vi "PostCopyScripting.vi"(10 "MetaDataObj":refnum<class "MetaDataObj.lvclass">, 11 "User Project":refnum<vi>) -> ()   [LabVIEW 2021, in "myRIOMetaDataObj.lvclass"]
uses:
  myRIOMetaDataObj.lvclass
  <resource>/dialog/NewProjectWizard/MetaDataObj/MetaDataObj.lvclass
  p:/lvdist/win32/export/21.0/21.0.0f0/dist/resource/dialog/NewProjectWizard/MetaDataObj/MetaDataObj.lvclass
  myRIOMetaDataObj.lvclass/myRIOMetaDataObj.ctl
  Read Target FPGA Personality.vi
  <resource>/dialog/NewProjectWizard/MetaDataObj/Accessors/Read Title.vi
  <vilib>/Utility/EditLVProj/Edit LVProj.lvlib
  <resource>/dialog/NewProjectWizard/Project Copying/NI_NPW_Project Copying.lvlib
  <vilib>/myRIO/Common/FPGA Personality Framework/Personality.lvlib
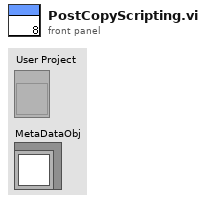
[diagram p1: front panel]
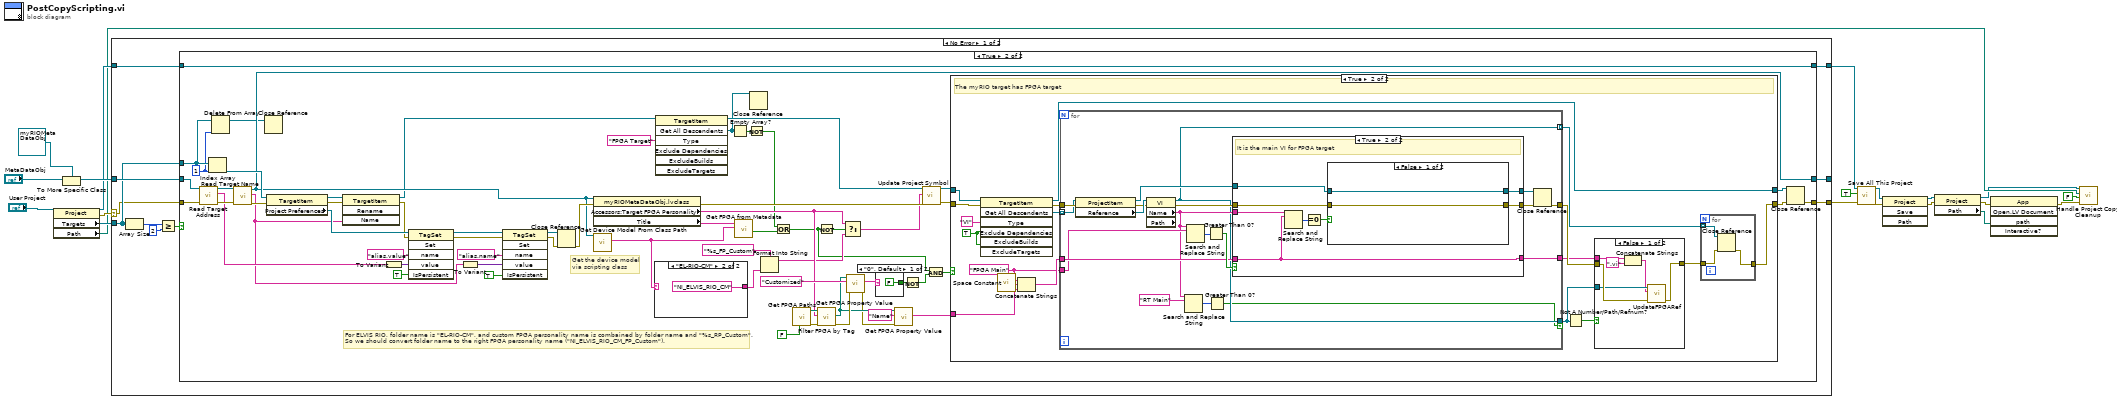
[diagram p0: block diagram]
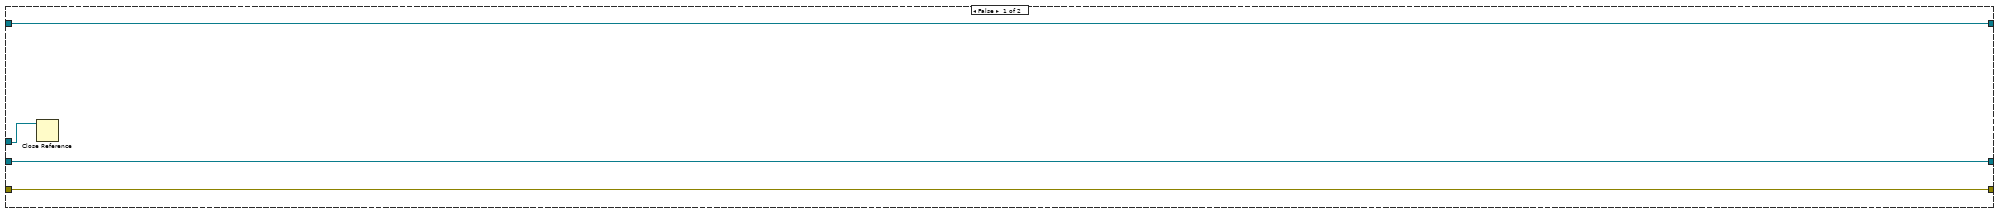
[diagram p2: hidden frame]
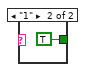
[diagram p4: hidden frame]
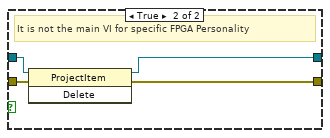
[diagram p8: hidden frame]
diagram:
  n1 = property class="Project"(reference="User Project") -> (reference out=w14:refnum<vi>, error out=w15:errorcluster, "Targets"=w16:refnum<vi>[], "Path"=w8:path)  [unwired: 1 in]
  n2 = To More Specific Class(target class=refnum<class "myRIOMetaDataObj.lvclass"> refnum ("myRIOMetaDataObj.lvclass"), reference="MetaDataObj") -> (specific class reference=w17:refnum<class "myRIOMetaDataObj.lvclass">)  [unwired: 1 in, 1 out]
  n3 = case shown="No Error" w15 {
    selector: w15 -> [w25 w169]
    tunnel: w17 -> [w27 w170]
    tunnel: w16 -> [w26 _]
    tunnel: [w24 w170] -> _
    tunnel: w14 -> [w22 w168]
    tunnel: [w23 w169] -> w13
    tunnel: [w21 w168] -> w12
    frame No Error {
      n4 = Array Size(array=w26) -> (size(s)=w30:i32)
      n5 = Greater Or Equal?(x=w30, y=2) -> (x >= y?=w28:bool)
      n6 = case shown="True" w28 {
        tunnel: w27 -> [w34 w94]
        tunnel: w26 -> [w31 w40]
        tunnel: w25 -> [w33 w93]
        tunnel: [w34 w62] -> w24
        tunnel: [w33 w85] -> w23
        tunnel: w22 -> [w32 w91]
        tunnel: [w32 w91] -> w21
        frame False {
          n7 = Close Reference(reference=w31) -> ()  [unwired: 1 in, 1 out]
        }
        frame True {
          w39 = 1 ("index")
          # "For ELVIS RIO, folder name is \"EL-RIO-CM\", and custom FPGA personality name is combained by folder name and \"%s_RP_Custom\".\nSo we should convert folder name to the right FPGA personality name (\"NI_ELVIS_RIO_CM_FP_Custom\")."
          # "Get the device model \nvia scripting class"
          n8 = call-dynamic "Read Target Address.vi"("error in (no error)"=w93, "myRIOMetaDataObj in"=w94) -> ("error out"=w65:errorcluster, "Target Address"=w61:string, "myRIOMetaDataObj out"=w63:refnum<class "myRIOMetaDataObj.lvclass">)  [unwired: 7 in]
          n9 = Index Array(array=w40, index=w39) -> (element=w97:refnum<vi>)
          n10 = Delete From Array(array=w40, index=w39) -> (array with subset deleted=w38:refnum<vi>[])  [unwired: 1 in, 1 out]
          n11 = call-dynamic "Read Target Name.vi"("error in (no error)"=w65, "myRIOMetaDataObj in"=w63) -> ("error out"=w64:errorcluster, "Target Name"=w48:string, "myRIOMetaDataObj out"=w62:refnum<class "myRIOMetaDataObj.lvclass">)  [unwired: 7 in]
          n12 = Close Reference(reference=w38) -> ()  [unwired: 1 in, 1 out]
          n13 = property class="TargetItem"(reference=w97, error in=w64) -> (reference out=w60:refnum<vi>, error out=w59:errorcluster, "Project Preferences"=w96:refnum<vi>)
          n14 = invoke class="TargetItem" method="Rename"(reference=w60, error in=w59, "Name"=w48) -> (reference out=w47:refnum<vi>, error out=w58:errorcluster)  [unwired: 1 in, 2 out]
          n15 = To Variant(anything=w61) -> (Variant=w92:variant)
          n16 = invoke class="TagSet" method="Set"(reference=w96, error in=w58, "name"="alias.value" ("Name"), "value"=w92, "IsPersistent"=TRUE ("Is Persistent")) -> (reference out=w56:refnum<vi>, error out=w53:errorcluster)  [unwired: 1 in, 4 out]
          n17 = To Variant(anything=w48) -> (Variant=w57:variant)
          n18 = invoke class="TagSet" method="Set"(reference=w56, error in=w53, "name"="alias.name" ("Name"), "value"=w57, "IsPersistent"=TRUE ("Is Persistent")) -> (reference out=w52:refnum<vi>, error out=w51:errorcluster)  [unwired: 1 in, 4 out]
          n19 = Close Reference(reference=w52, error in (no error)=w51) -> (error out=w87:errorcluster)
          n20 = property class="myRIOMetaDataObj.lvclass"(reference=w62, error in=w87) -> (error out=w90:errorcluster, "Accessors:Target FPGA Personality"=w75:string, "Title"=w82:string)  [unwired: 1 out]
          n21 = call "Get Device Model From Class Path.vi"("MetaDataObj in"=w62) -> ("Device Model Str"=w36:string)  [unwired: 8 in, 2 out]
          n22 = case shown="\"EL-RIO-CM\"" w36 {
            selector: w36 -> [w98 _]
            tunnel: [w98 "NI_ELVIS_RIO_CM"] -> w35
            frame Default {
            }
            frame "EL-RIO-CM" {
            }
          }
          n23 = invoke class="TargetItem" method="Get All Descendents"(reference=w47, "Type"="FPGA Target") -> (reference out=w46:refnum<vi>, "All Descendents"=w37:refnum<vi>[])  [unwired: 5 in, 5 out]
          n24 = Empty Array?(array=w37) -> (empty?=w41:bool)
          n25 = call <vilib>:"Get FPGA from Metadata.vi"("Device Model Str"=w36, "Title"=w82) -> ("Customized?"=w43:bool)  [unwired: 5 in, 4 out]
          n26 = Not(x=w41) -> (.not. x?=w44:bool)
          n27 = Close Reference(reference=w37) -> ()  [unwired: 1 in, 1 out]
          n28 = Format Into String(format string="%s_FP_Custom" ("Target FPGA Personality"), w35) -> (resulting string=w49:string)  [unwired: 2 in, 1 out]
          n29 = Or(x=w44, y=w43) -> (x .or. y?=w42:bool)
          n30 = call <vilib>:"Get FPGA Paths.vi"("Filter Customized (T)"=FALSE) -> ("error out"=w79:errorcluster, "FPGA Personality File Paths"=w78:path[])  [unwired: 9 in]
          n31 = Not(x=w42) -> (.not. x?=w71:bool)
          n32 = call <vilib>:"Filter FPGA by Tag.vi"("error in (no error)"=w79, "FPGA Personality Tag"=w75, "FPGA Personality File Paths"=w78) -> ("error out"=w70:errorcluster, "First Path"=w69:path)  [unwired: 6 in, 1 out]
          n33 = Select(t=w75, s=w71, f=w49) -> (s? t:f=w81:string)
          n34 = call <vilib>:"Get FPGA Property Value.vi"("error in (no error)"=w70, "Property Name"="Customized" ("Target FPGA Personality"), "FPGA Personality File Path"=w69) -> ("error out"=w67:errorcluster, "Property Value"=w74:string)  [unwired: 5 in, 2 out]
          n35 = case shown="\"0\", Default" w74 {
            tunnel: [FALSE ("Filter Customized (T)") TRUE ("Filter Customized (T)")] -> w73
            frame "0", Default {
            }
            frame "1" {
            }
          }
          n36 = call <vilib>:"Get FPGA Property Value.vi"("error in (no error)"=w67, "Property Name"="Name", "FPGA Personality File Path"=w69) -> ("Property Value"=w66:string)  [unwired: 5 in, 3 out]
          n37 = Not(x=w73) -> (.not. x?=w72:bool)
          n38 = call <vilib>:"Update Project Symbol.vi"("error in (no error)"=w90, "New FPGA Personality Value"=w81, "TargetItem Refnum"=w46) -> ("error out"=w89:errorcluster, "Duplicated TargetItem Refnum"=w80:refnum<vi>)  [unwired: 7 in]
          n39 = And(x=w42, y=w72) -> (x .and. y?=w83:bool)
          n40 = case shown="True" w83 {
            tunnel: w89 -> [w103 w119]
            tunnel: [w103 w105] -> w86
            tunnel: w80 -> [w102 w116]
            tunnel: w66 -> [_ w113]
            tunnel: [w102 w109] -> w84
            frame False {
            }
            frame True {
              w112 = "FPGA Main" ("search string")
              w120 = TRUE ("ExcludeDependencies")
              # "The myRIO target has FPGA target"
              n41 = invoke class="TargetItem" method="Get All Descendents"(reference=w116, error in=w119, "Type"="VI", "Exclude Dependencies"=w120, "ExcludeBuilds"=w120) -> (reference out=w109:refnum<vi>, error out=w118:errorcluster, "All Descendents"=w117:refnum<vi>[])  [unwired: 2 in, 4 out]
              n42 = call <vilib>:"Space Constant.vi"() -> ("String"=w115:string)
              n43 = Concatenate Strings(w112, w115, w113) -> (w114:string)
              n44 = for {
                tunnel: w118 -> [w150]
                tunnel: w117 -> [w149] mode=indexing
                tunnel: w114 -> [w145]
                tunnel: [w140] -> w110
                tunnel: w112 -> [w139]
                tunnel: [w134] -> w108
                tunnel: [w133] -> w107 mode=indexing
                tunnel: [w133] -> w104 if=w132
                n45 = property class="ProjectItem"(reference=w149, error in=w150) -> (reference out=w143:refnum<vi>, error out=w144:errorcluster, "Reference"=w148:refnum<vi>)
                n46 = property class="VI" props=["Name", "Path"](reference=w148, error in=w144) -> (reference out=w133:refnum<vi>, error out=w135:errorcluster, "Name"=w138:string)  [unwired: 1 out]
                n47 = Search and Replace String(input string=w138, search string="RT Main") -> (number of replacements=w137:i32)  [unwired: 6 in, 3 out]
                n48 = Search and Replace String(input string=w138, search string=w139) -> (number of replacements=w147:i32)  [unwired: 6 in, 3 out]
                n49 = Greater Than 0?(x=w147) -> (x > 0?=w146:bool)
                n50 = Greater Than 0?(x=w137) -> (x > 0?=w132:bool)
                n51 = case shown="True" w146 {
                  tunnel: w145 -> [w151 w154]
                  tunnel: w138 -> [_ w161]
                  tunnel: w143 -> [w153 w158]
                  tunnel: w135 -> [w152 w157]
                  tunnel: [w152 w156] -> w141
                  tunnel: [w153 w155] -> w142
                  tunnel: [w151 w154] -> w134
                  frame False {
                  }
                  frame True {
                    # "It is the main VI for FPGA target"
                    n52 = Search and Replace String(input string=w161, search string=w154) -> (number of replacements=w160:i32)  [unwired: 6 in, 3 out]
                    n53 = Equal To 0?(x=w160) -> (x = 0?=w159:bool)
                    n54 = case shown="False" w159 {
                      tunnel: w158 -> [w162 w167]
                      tunnel: w157 -> [w163 w166]
                      tunnel: [w163 w165] -> w156
                      tunnel: [w162 w164] -> w155
                      frame False {
                      }
                      frame True {
                        # "It is not the main VI for specific FPGA Personality"
                        n55 = invoke class="ProjectItem" method="Delete"(reference=w167, error in=w166) -> (reference out=w164:refnum<vi>, error out=w165:errorcluster)  [unwired: 1 in, 1 out]
                      }
                    }
                  }
                }
                n56 = Close Reference(reference=w142, error in (no error)=w141) -> (error out=w140:errorcluster)
              }
              n57 = Not A Number/Path/Refnum?(number/path/refnum=w104) -> (NaN/Path/Refnum?=w111:bool)
              n58 = case shown="False" w111 {
                tunnel: w110 -> [w130 w131]
                tunnel: [w128 w131] -> w106
                tunnel: w104 -> [w129 _]
                tunnel: w108 -> [w126 _]
                frame False {
                  n59 = Concatenate Strings(w126, ".vi" ("string")) -> (w127:string)
                  n60 = call "UpdateFPGARef.vi"("error in (no error)"=w130, "FPGA Target Main VI"=w127, "VI Refnum"=w129) -> ("error out"=w128:errorcluster)  [unwired: 7 in, 1 out]
                }
                frame True {
                }
              }
              n61 = for {
                tunnel: w107 -> [w124] mode=indexing
                tunnel: w106 -> [w123]
                tunnel: [w122] -> w105
                n62 = Close Reference(reference=w124, error in (no error)=w123) -> (error out=w122:errorcluster)
              }
            }
          }
          n63 = Close Reference(reference=w84, error in (no error)=w86) -> (error out=w85:errorcluster)
        }
      }
    }
    frame Error {
    }
  }
  n64 = call <vilib>:"Save All This Project.vi"("error in (no error)"=w13, "Exclude Dependencies? (F)"=TRUE, "Project in"=w12) -> ("error out"=w9:errorcluster, "Project out"=w10:refnum<vi>)  [unwired: 7 in]
  n65 = invoke class="Project" method="Save"(reference=w10, error in=w9) -> (reference out=w4:refnum<vi>, error out=w5:errorcluster)  [unwired: 2 in, 2 out]
  n66 = property class="Project"(reference=w4, error in=w5) -> (reference out=w1:refnum<vi>, error out=w3:errorcluster, "Path"=w2:path)
  n67 = invoke class="App" method="Open.LV Document"(error in=w3, "path"=w2) -> (error out=w7:errorcluster)  [unwired: 3 in, 4 out]
  n68 = call <resource>:"Handle Project Copy Cleanup.vi"("error in (no error)"=w7, "More Scripting?"=FALSE, "Target Path"=w8, "Project in"=w1) -> ()  [unwired: 8 in]
